vi "FingerThreshold.vi"(2 "Threshold":dbl, 3 "task/channels in":refnum<k21>) -> (0 "FingerPos":dbl, 1 "FingerStatus":enum16{"Above Threshold", "Below Threshold"}(ring))   [LabVIEW 2011]
uses:
  <vilib>/DAQmx/read.llb/DAQmx Read (Counter DBL 1Chan 1Samp).vi
  <vilib>/DAQmx/miscellaneous.llb/DAQmx Fill In Error Info.vi
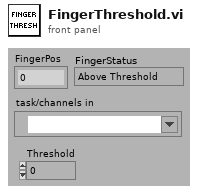
[diagram p1: front panel]
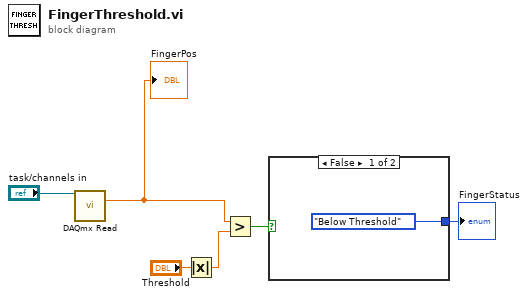
[diagram p0: block diagram]
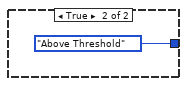
[diagram p2: hidden frame]
diagram:
  n1 = call-poly <vilib>:"DAQmx Read.vi"("task/channels in"="task/channels in") -> ("data"=w4:dbl)  [unwired: 12 in, 2 out]
  "FingerPos" <- w4
  n2 = Absolute Value(x="Threshold") -> (abs(x)=w1:dbl)
  n3 = Greater?(x=w4, y=w1) -> (0:w5:bool)
  n4 = case shown="False" w5 {
    tunnel: [enum16{"Above Threshold", "Below Threshold"}."Below Threshold" ("Index") enum16{"Above Threshold", "Below Threshold"}."Above Threshold" ("Index")] -> w3
    frame False {
    }
    frame True {
    }
  }
  "FingerStatus" <- w3
